vi "Actor Core.vi"(8 "error in":errorcluster, 11 "startconteo in":refnum<class "startconteo.lvclass">) -> (0 "error out":errorcluster, 3 "Actor out":refnum<class "Actor.lvclass">)   [LabVIEW 2019, in "startconteo.lvlib" / "startconteo.lvclass"]
doc: "(<B>Filename</B>: Actor Framework.lvlib:Actor.lvclass:Actor Core.vi)\n\nReceives messages to the actor, reacts to them, and initiates any error handling that may shut the actor down.\n\nDescendant classes may override this VI to append parallel tasks for the actor to complete while it handles messages. Overrides use the Call Parent Method node."
uses:
  startconteo.lvclass
  C:/Program Files (x86)/National Instruments/LabVIEW 2019/vi.lib/ActorFramework/Actor/Actor.lvclass
  <vilib>/ActorFramework/Actor/Actor.lvclass
  <vilib>/ActorFramework/Actor/Actor.lvclass/Actor.ctl
  startconteo.lvclass/startconteo.ctl
  ContadorB Messages/contar Msg/contar Msg.lvclass/contar Msg.ctl
  <vilib>/ActorFramework/Message Enqueuer/Message Enqueuer.lvclass/Message Enqueuer.ctl
  <vilib>/ActorFramework/Message Enqueuer/Enqueue.vi
  ContadorB Messages/contar Msg/contar Msg.lvclass
  C:/Program Files (x86)/National Instruments/LabVIEW 2019/vi.lib/ActorFramework/Message/Message.lvclass
  <vilib>/ActorFramework/Message Priority Queue/Priority Enqueue.vi
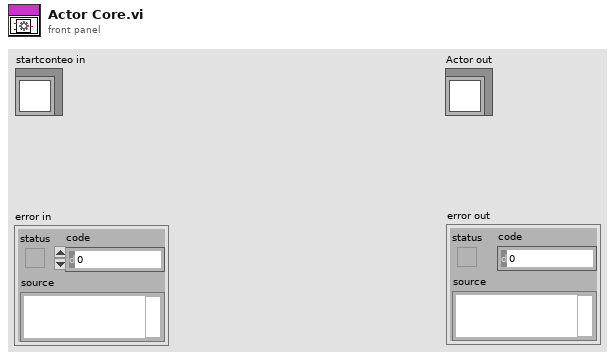
[diagram p1: front panel]
types:
  T1 = cluster{"StartStop HL":refnum<user-event>, "Exit":refnum<user-event>, "Maximo":refnum<user-event>}
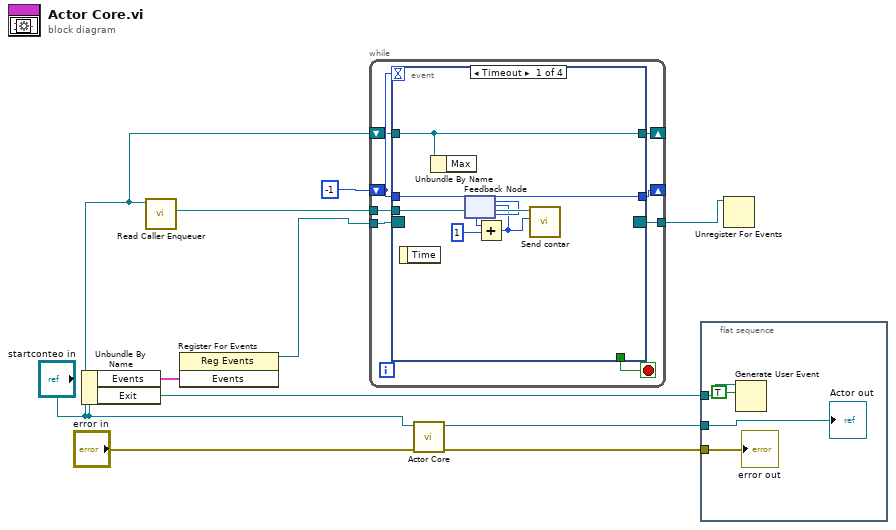
[diagram p0: block diagram]
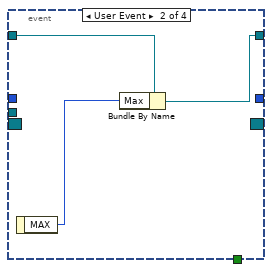
[diagram p2: hidden frame]
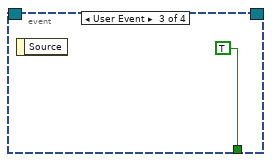
[diagram p3: hidden frame]
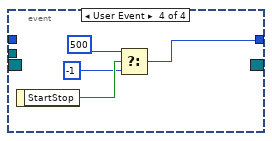
[diagram p4: hidden frame]
diagram:
  n1 = Unbundle By Name("startconteo in") -> ("Events"=w6:T1, "Exit"=w2:refnum<user-event>)
  n2 = call <vilib>:"Read Caller Enqueuer.vi"("Actor"="startconteo in") -> ("Caller Enqueuer"=w3:refnum<class "Message Enqueuer.lvclass">)  [unwired: 10 in]
  n3 = register-events(w6) -> (reference out=w5:refnum<event-registration>)  [unwired: 2 in, 1 out]
  n4 = while {
    shift-right: [w17] -> _
    shift-left: -1 -> [w18]
    tunnel: w5 -> [w16]
    tunnel: [w15] -> w4
    tunnel: w3 -> [w13]
    shift-right: [w12] -> _
    shift-left: "startconteo in" -> [w11]
    stop <- w14 stop-if-true
    n5 = event shown="[0] Timeout" {
      selector: w16 -> [_ _ _ _]
      dyn-events: [_ _ _ _] -> w15
      timeout: w18 -> [_ _ _ _]
      tunnel: w18 -> [w24 _ _ _]
      tunnel: [w24 _ _ w29] -> w17
      tunnel: [_ _ TRUE _] -> w14
      tunnel: w13 -> [w23 _ _ _]
      tunnel: [w19 w26 _ _] -> w12
      tunnel: w11 -> [w19 w27 _ _]
      event Timeout {
        n6 = event-data() -> ()  [unwired: 1 in, 1 out]
        n7 = Unbundle By Name(w19) -> ()  [unwired: 1 out]
        n8 = feedback #1() -> (w21:i32)  [unwired: 1 in]
        n9 = Add(x=w21, y=1) -> (x+y=w20:i32)
        n10 = feedback-in #1(w20) -> ()
        n11 = call "Send contar.vi"("Cuenta"=w20, "Message Enqueuer"=w23) -> ()  [unwired: 8 in, 2 out]
      }
      event User Event {
        n12 = event-data() -> ("MAX"=w25:i32)  [unwired: 1 in]
        n13 = Bundle By Name(cluster=w27, "Max"=w25) -> (w26:refnum<class "startconteo.lvclass">)
      }
      event User Event {
        n14 = event-data() -> ()  [unwired: 1 in, 1 out]
      }
      event User Event {
        n15 = event-data() -> ("StartStop"=w32:bool)  [unwired: 1 in]
        n16 = Select(t=500, s=w32, f=-1) -> (s? t:f=w29:i32)
      }
    }
  }
  n17 = call-parent "Actor Core.vi"("error in"="error in", "Actor in"="startconteo in") -> ("error out"=w10:errorcluster, "Actor out"=w9:refnum<class "Actor.lvclass">)  [unwired: 8 in]
  n18 = flat-sequence {
    tunnel: w10 -> [w36]
    tunnel: w9 -> [w35]
    tunnel: w2 -> [w34]
    frame #0 {
      n19 = Generate User Event(user event=w34, event data cluster=TRUE ("event data")) -> ()  [unwired: 2 in, 2 out]
      "error out" <- w36
      "Actor out" <- w35
    }
  }
  n20 = Unregister For Events(event registration refnum=w4) -> ()  [unwired: 1 in, 1 out]
